vi "PCO_SetIntensifiedGatingMode.vi"(8 "error in (no error)":errorcluster {"code" format="%x"}, 10 "wIntensifiedGatingMode":u16, 11 "ph":u64) -> (0 "error out":errorcluster {"code" format="%x"}, 2 "ErrorMessage":i32 format="%x", 3 "ph out":u64)   [LabVIEW 2020, in "SDK.lvlib" / "SpecialCommandsDicam.lvlib"]
doc: "SC2_SDK_FUNC int WINAPI PCO_SetIntensifiedGatingMode(HANDLE ph,\n WORD wIntensifiedGatingMode,\n WORD wReserved);"
uses:
  SpecialCommandsDicam.lvlib
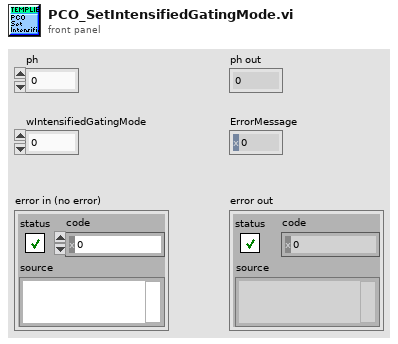
[diagram p1: front panel]
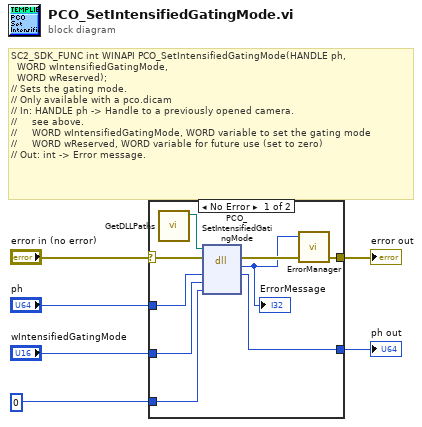
[diagram p0: block diagram]
diagram:
  # "SC2_SDK_FUNC int WINAPI PCO_SetIntensifiedGatingMode(HANDLE ph,\n  WORD wIntensifiedGatingMode,\n  WORD wReserved);\n// Sets the gating mode.\n// Only available with a pco.dicam\n// In: HANDLE ph -> Handle to a previously opened camera.\n//     see above.\n//     WORD wIntensifiedGatingMode, WORD variable to set the gating mode\n//     WORD wReserved, WORD variable for future use (set to zero)\n// Out: int -> Error message."
  n1 = case shown="No Error" "error in (no error)" {
    selector: "error in (no error)" -> [w11 w17]
    tunnel: "ph" -> [w15 w16]
    tunnel: [w14 w16] -> w5
    tunnel: "wIntensifiedGatingMode" -> [w13 _]
    tunnel: [w10 w17] -> w3
    tunnel: u16 0 ("wReserved") -> [w12 _]
    frame No Error {
      n2 = call "GetDLLPaths.vi"() -> ("SC2_Cam_Path"=w7:path)  [unwired: 9 in, 2 out]
      n3 = dll-call lib="?" fn="PCO_SetIntensifiedGatingMode"(path in=w7, error in=w11, "ph"=w15, "wIntensifiedGatingMode"=w13, "wReserved"=w12) -> (error out=w9:errorcluster, "return type"=w8:i32, "ph"=w14:u64)  [unwired: 3 in, 1 out]
      "ErrorMessage" <- w8
      n4 = call "ErrorManager.vi"("error in (no error)"=w9, "error code"=w8) -> ("error out"=w10:errorcluster)  [unwired: 3 in]
    }
    frame Error {
    }
  }
  "ph out" <- w5
  "error out" <- w3
